vi "Emergency Stop.vi"(8 "error in (no error)":errorcluster, 11 "Protected Actor Handle in":refnum<class "Protected Actor Handle.lvclass">) -> (0 "error out":errorcluster)   [LabVIEW 2020, in "AF Debug.lvlib" / "Protected Actor Handle.lvclass"]
doc: "Sends the Stop Msg to the actor with emergency priority."
uses:
  Protected Actor Handle.lvclass
  Protected Actor Handle.lvclass/Protected Actor Handle.ctl
  vi.lib/ActorFramework/Inspection API/Protected Actor Handle/Protected Actor Handle.lvclass
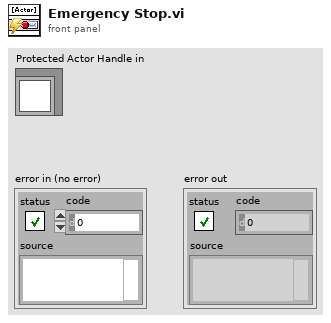
[diagram p1: front panel]
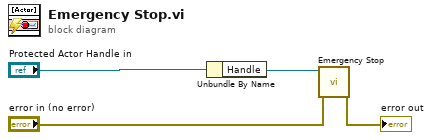
[diagram p0: block diagram]
diagram:
  n1 = Unbundle By Name("Protected Actor Handle in") -> ("Handle"=w1:refnum<class "Protected Actor Handle.lvclass">)
  n2 = call "Emergency Stop.vi"("error in (no error)"="error in (no error)", "Protected Actor Handle in"=w1) -> ("error out"=→"error out":errorcluster)  [unwired: 9 in]
